vi "find.folders.with.missing.issues.vi"() -> ()   [LabVIEW 2024]
panel:
  out "iteration":i32
  out "currrent folder":string
  out "Array":string[](array[string])
  out "error out":errorcluster
  in  "Folder Path":path=path "D:/Comics/Marvel"
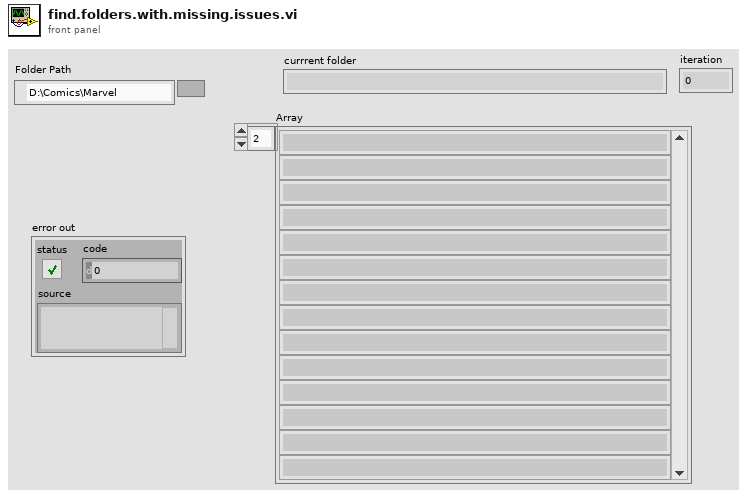
[diagram p1: front panel]
types:
  T1 = typedef "comics.reply--cluster.ctl" = cluster{"code":i32, "status":string, "etag":string, "data":cluster{"offset":i32, "limit":i32, "total":i32, "count":i32, "results":T2[]}}
  T2 = typedef "comic--cluster.ctl" = cluster{"id":i32, "digitalId":i32, "title":string, "issueNumber":i32, "variantDescription":string, "description":string, "modified":variant, "upc":string, "format":string, "pageCount":i32, "resourceURI":string, "urls":cluster{"type":string, "url":string}[], "series":cluster{"resourceURI":string, "name":string}, "dates":cluster{"type":string, "date":string}[], "prices":cluster{"price":dbl, "type":string}[], "thumbnail":cluster{"path":string, "extension":string}, "images":cluster{"path":string, "extension":string}[], "creators":cluster{"available":i32, "returned":i32, "collectionURI":string, "items":cluster{"resourceURI":string, "name":string, "role":string}[]}, "characters":cluster{"available":i32, "returned":i32, "collectionURI":string, "items":cluster{"resourceURI":string, "name":string}[]}, "stories":cluster{"available":i32, "returned":i32, "collectionURI":string, "items":cluster{"resourceURI":string, "name":string, "type":string}[]}, "events":cluster{"available":i32, "returned":i32, "collectionURI":string, "items":cluster{"resourceURI":string, "name":string}[]}}
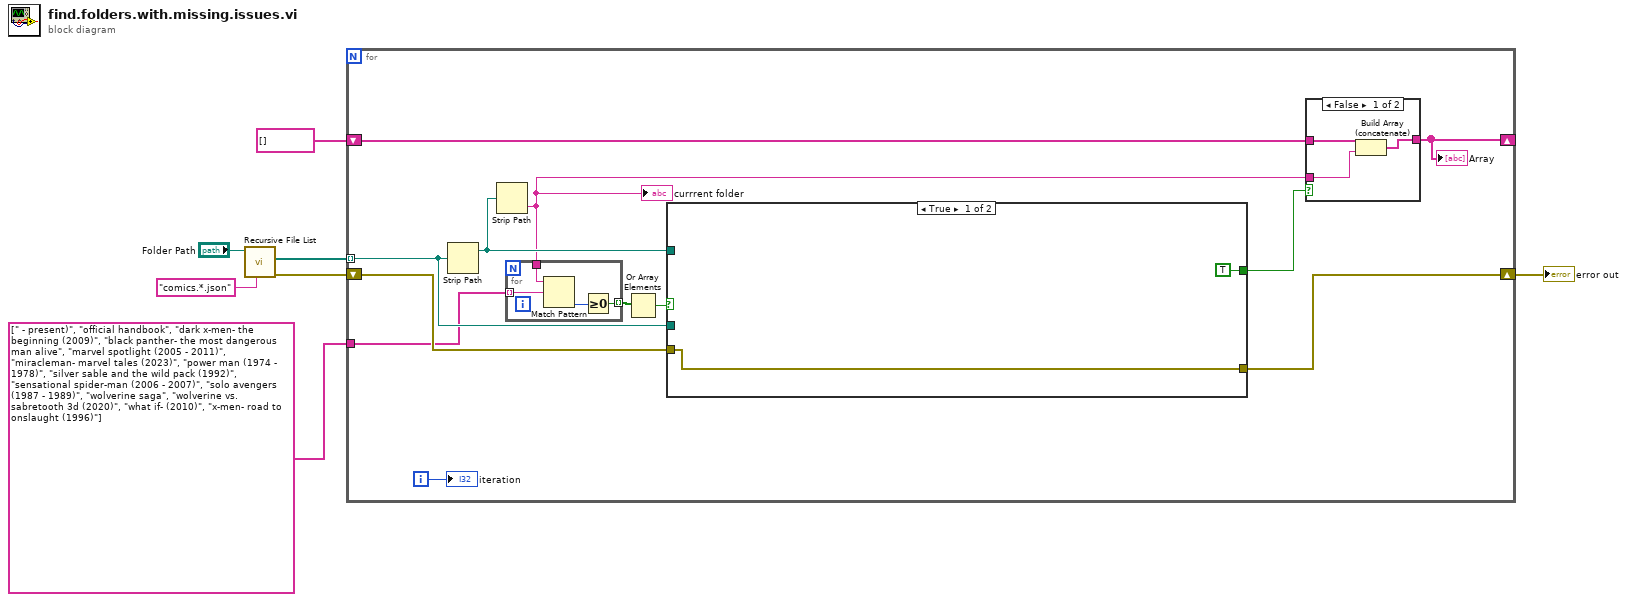
[diagram p0: block diagram]
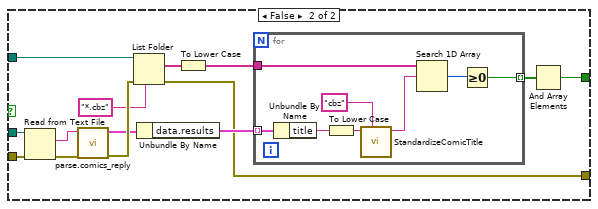
[diagram p2: hidden frame]
diagram:
  n1 = call <vilib>:"Recursive File List.vi"("pattern"="comics.*.json", "Folder Path"="Folder Path") -> ("error out"=w4:errorcluster, "All Files in Dir"=w5:path[])  [unwired: 5 in, 3 out]
  n2 = for {
    tunnel: w5 -> [w17] mode=indexing
    shift-right: [w12] -> w3
    shift-left: w4 -> [w16]
    shift-right: [w13] -> _
    shift-left: string[] [] -> [w19]
    tunnel: string[] [" - present)", "official handbook", "dark x-men- the beginning (2009)", "black panther- the most dangerous man alive", "marvel spotlight (2005 - 2011)", "miracleman- marvel tales (2023)", "power man (1974 - 1978)", "silver sable and the wild pack (1992)", "sensational spider-man (2006 - 2007)", "solo avengers (1987 - 1989)", "wolverine saga", "wolverine vs. sabretooth 3d (2020)", "what if- (2010)", "x-men- road to onslaught (1996)"] -> [w10]
    i -> [w18]
    n3 = Strip Path(path=w17) -> (stripped path=w14:path)  [unwired: 1 out]
    n4 = Strip Path(path=w14) -> (name=w11:string)  [unwired: 1 out]
    "currrent folder" <- w11
    n5 = for {
      tunnel: w11 -> [w23]
      tunnel: w10 -> [w22] mode=indexing
      tunnel: [w20] -> w8 mode=indexing
      n6 = Match Pattern(string=w23, regular expression=w22) -> (offset past match=w21:i32)  [unwired: 1 in, 3 out]
      n7 = Greater Or Equal To 0?(x=w21) -> (x >= 0?=w20:bool)
    }
    n8 = Or Array Elements(Boolean array=w8) -> (logical OR=w9:bool)
    n9 = case shown="True" w9 {
      tunnel: w17 -> [_ w37]
      tunnel: w16 -> [w24 w36]
      tunnel: [TRUE w30] -> w15
      tunnel: w14 -> [_ w29]
      tunnel: [w24 w28] -> w12
      frame True {
      }
      frame False {
        n10 = Read from Text File(file (use dialog)=w37, error in=w36) -> (text=w38:string, error out=w39:errorcluster)  [unwired: 2 in, 2 out]
        n11 = call "parse.comics_reply.vi"("error in"=w39, "string in"=w38) -> ("error out"=w35:errorcluster, "data"=w34:T1)  [unwired: 8 in]
        n12 = List Folder(path=w29, pattern="*.cbz", error in=w35) -> (filenames=w26:string[], error out=w28:errorcluster)  [unwired: 1 in, 2 out]
        n13 = Unbundle By Name(w34) -> ("data.results"=w33:T2[])
        n14 = To Lower Case(string=w26) -> (all lower case string=w27:string[])
        n15 = for {
          tunnel: w33 -> [w47] mode=indexing
          tunnel: w27 -> [w46]
          tunnel: [w44] -> w31 mode=indexing
          n16 = Unbundle By Name(w47) -> ("title"=w43:string)
          n17 = To Lower Case(string=w43) -> (all lower case string=w42:string)
          n18 = call "StandardizeComicTitle.vi"("extention (\"\"=none)"="cbz" ("extention (\"\"=none)"), "title in"=w42) -> ("title out"=w40:string)  [unwired: 9 in]
          n19 = Search 1D Array(1D array=w46, element=w40) -> (index of element=w45:i32)  [unwired: 1 in]
          n20 = Greater Or Equal To 0?(x=w45) -> (x >= 0?=w44:bool)
        }
        n21 = And Array Elements(Boolean array=w31) -> (logical AND=w30:bool)
      }
    }
    n22 = case shown="False" w15 {
      tunnel: w19 -> [w50 w51]
      tunnel: [w49 w51] -> w13
      tunnel: w11 -> [w48 _]
      frame False {
        n23 = Build Array (concatenate)(w50, w48) -> (w49:string[])
      }
      frame True {
      }
    }
    "Array" <- w13
    "iteration" <- w18
  }
  "error out" <- w3
